vi "Trigger AI Acquisition.vi"() -> ()   [LabVIEW 2012]
doc: "This example demonstrates how to continuously acquire buffered voltage measurements using a DAQmx device.\n\nFor instructions on how to connect your signals to the DAQ device, refer to your device documentation."
uses:
  <resource>/objmgr/daqmx.rc
  <vilib>/DAQmx/configure/trigger.llb/DAQmx Start Trigger (Digital Edge).vi
  <vilib>/DAQmx/read.llb/DAQmx Read (Analog 1D Wfm NChan NSamp).vi
  <vilib>/DAQmx/configure/task.llb/DAQmx Configure Logging (TDMS).vi
  <vilib>/DAQmx/configure/timing.llb/DAQmx Timing (Sample Clock).vi
  <vilib>/DAQmx/create/channels.llb/DAQmx Create Channel (AI-Voltage-Basic).vi
panel:
  in  "edge":i32(ring)=10280 items=["Rising"=10280, "Falling"=10171]
  in  "source":tag="/Dev1/PFI1"
  in  "Stop":bool
  out "Waveform Graph":waveform(dbl)[](graph)=[{"t0"=timestamp(3423073651.7132955 s since 1904-01-01), "dt"=0.001, "Y"=array[1000 elements], "attributes"=variant("NI_ChannelName"=variant(string "Dev1/ai1"), "NI_UnitDescription"=variant(string "Volts"))}]
  in  "TDMS File Path":path
  in  "Samples per Loop":i32=1000
  in  "Sample Rate":dbl=1000.0
  in  "Sample Clock Source":tag="OnboardClock"
  in  "Terminal Configuration":i32(ring)=-1 items=["default"=-1, "RSE"=10083, "NRSE"=10078, "Differential"=10106, "Pseudodifferential"=12529]
  in  "Max Voltage":dbl=1.0
  in  "Min Voltage":dbl=-1.0
  in  "Physical Channel":tag="Dev1/ai1"
  out "Actual Sample Rate":dbl=1000.0 format="%0.2f"
  in  "Logging Mode":i32(ring)=10231 items=["Off"=10231, "Log and Read"=15842]
  # "Channel Settings"
  # "Trigger Settings"
  # "Acquired Data"
  # "Timing Settings"
  # "Logging Settings"
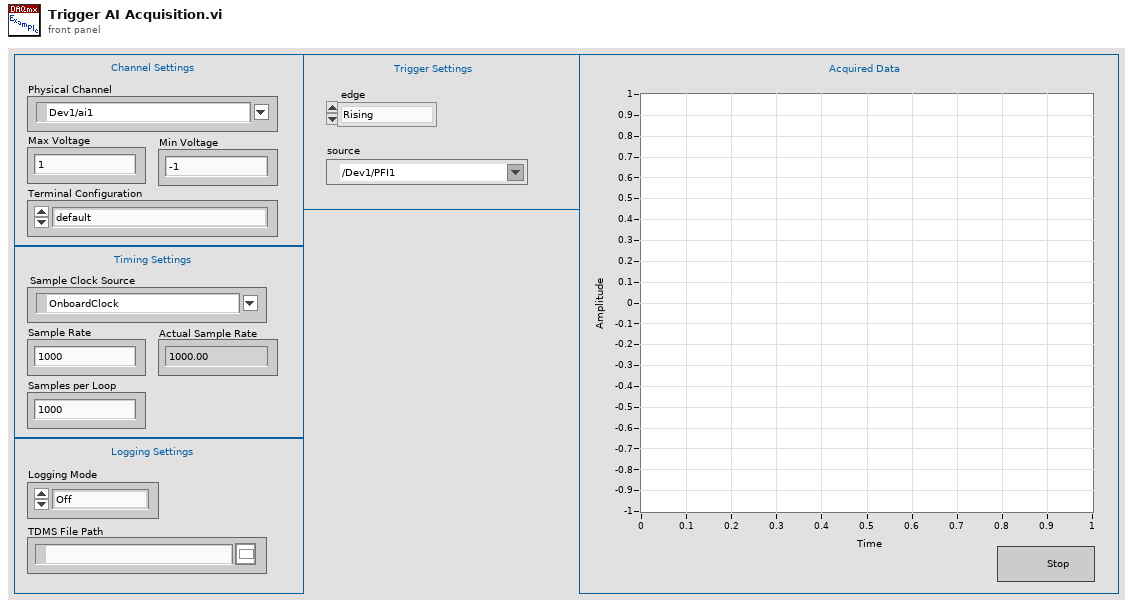
[diagram p1: front panel]
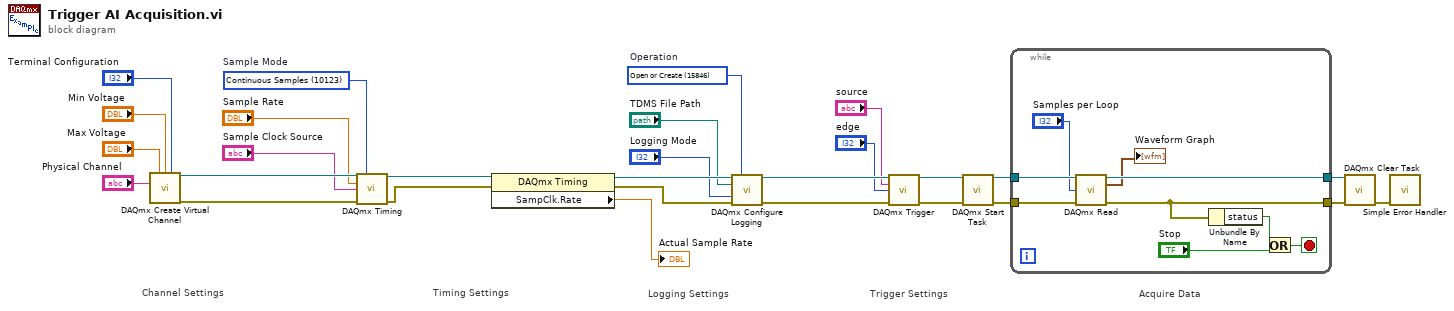
[diagram p0: block diagram]
diagram:
  w21 = 15846 items=["Open"=10437, "Open or Create"=15846, "Create or Replace"=15847, "Create"=15848]  # Operation
  w26 = 10123 items=["Finite Samples"=10178, "Continuous Samples"=10123, "Hardware Timed Single Point"=12522]  # Sample Mode
  # "Trigger Settings"
  # "Acquire Data"
  # "Timing Settings"
  # "Channel Settings"
  # "Logging Settings"
  n1 = call-poly <vilib>:"DAQmx Create Virtual Channel.vi"("maximum value"="Max Voltage", "minimum value"="Min Voltage", "input terminal configuration"="Terminal Configuration", "physical channels"="Physical Channel") -> ("task out"=w24:refnum<k21>, "error out"=w25:errorcluster)  [unwired: 10 in]
  n2 = call-poly <vilib>:"DAQmx Timing.vi"("task/channels in"=w24, "sample mode"=w26, "rate"="Sample Rate", "source"="Sample Clock Source", "error in"=w25) -> ("task out"=w28:refnum<k21>, "error out"=w27:errorcluster)  [unwired: 9 in]
  n3 = property class="DAQmx Timing"(reference=w28, error in=w27) -> (reference out=w23:refnum<k21>, error out=w22:errorcluster, "SampClk.Rate"=→"Actual Sample Rate":dbl)
  n4 = call-poly <vilib>:"DAQmx Configure Logging.vi"("task/channels in"=w23, "operation"=w21, "file path"="TDMS File Path", "logging mode"="Logging Mode", "error in"=w22) -> ("task out"=w6:refnum<k21>, "error out"=w4:errorcluster)  [unwired: 9 in]
  n5 = call-poly <vilib>:"DAQmx Trigger.vi"("task/channels in"=w6, "source"="source", "edge"="edge", "error in"=w4) -> ("task out"=w5:refnum<k21>, "error out"=w3:errorcluster)  [unwired: 10 in]
  n6 = call <vilib>:"DAQmx Start Task.vi"("task/channels in"=w5, "error in"=w3) -> ("task out"=w20:refnum<k21>, "error out"=w19:errorcluster)  [unwired: 12 in]
  n7 = while {
    tunnel: w20 -> [w37]
    tunnel: w19 -> [w36]
    tunnel: [w33] -> w17
    tunnel: [w34] -> w18
    stop <- w35 stop-if-true
    n8 = call-poly <vilib>:"DAQmx Read.vi"("task/channels in"=w37, "number of samples per channel"="Samples per Loop", "error in"=w36) -> ("task out"=w34:refnum<k21>, "data"=→"Waveform Graph":waveform(dbl)[], "error out"=w33:errorcluster)  [unwired: 10 in]
    n9 = Unbundle By Name(w33) -> ("status"=w32:bool)
    n10 = Or(x=w32, y="Stop") -> (x .or. y?=w35:bool)
  }
  n11 = call <vilib>:"DAQmx Clear Task.vi"("task in"=w18, "error in"=w17) -> ("error out"=w16:errorcluster)  [unwired: 13 in]
  n12 = call <vilib>:"Simple Error Handler.vi"("error in (no error)"=w16) -> ()  [unwired: 4 in, 5 out]
